vi "Host.vi"() -> ()   [LabVIEW 2019]
uses:
  <vilib>/Utility/Variable/NI_VariableUtilities.lvlib
  <vilib>/Utility/file.llb/Write Delimited Spreadsheet (DBL).vi
  <vilib>/Utility/file.llb/Read Delimited Spreadsheet (DBL).vi
panel:
  out "Rounds":i32
  in  "Load Path":bool
  in  "Save Path":bool
  out "z ls error":T1
  out "z en error":T1
  out "x ls error":T1
  out "x en error":T1
  in  "tLength":i32=15000
  in  "t0":i32=7500
  out "X LS (mm)":dbl[](graph)
  out "Z LS (mm)":dbl[](graph)
  out "LS Error X  (um)":dbl[](graph)
  out "EN Error X  (um)":dbl[](graph)
  out "LS Error Z  (um)":dbl[](graph)
  out "EN Error Z  (um)":dbl[](graph)
  in  "Save 2 txt":bool caption="Save ILC"
  out "Z EN (mm)":dbl[](graph)
  out "X EN (mm)":dbl[](graph)
  in  "Load data":bool caption="Save ILC"
  in  "Stop Host":bool
  in  "Generate Path":bool
  out "Position Command X (mm)":dbl[](graph)
  out "Position Command Z (mm)":dbl[](graph)
  in  "CLEAR X":bool
  in  "CLEAR Z":bool
  in  "ADD X":bool
  in  "ADD Z":bool
  in  "Time (s)":dbl=30.0 format="%#_13g"
  in  "Sample Rate (Hz)":dbl=1000.0 format="%#_13g"
  in  "Tab Control":enum32{"Const", "Ramp", "Chirp", "Sin", "Cos"}(tab)
  in  "Constant Value (mm)":dbl format="%#_13g"
  in  "Ramp Value (mm)":dbl=-10.0 format="%#_13g"
  in  "Chirp  Amp (mm)":dbl=50.0
  in  "Initial Frequency (Hz)":dbl
  in  "Final Frequency (Hz)":dbl=50.0
  in  "Decay":bool=TRUE
  in  "Sin  Amp (mm)":dbl=-50.0
  in  "Sin Periods (s)":dbl=15.0
  in  "Cos  Amp (mm)":dbl=50.0
  in  "Cos Periods (s)":dbl=15.0
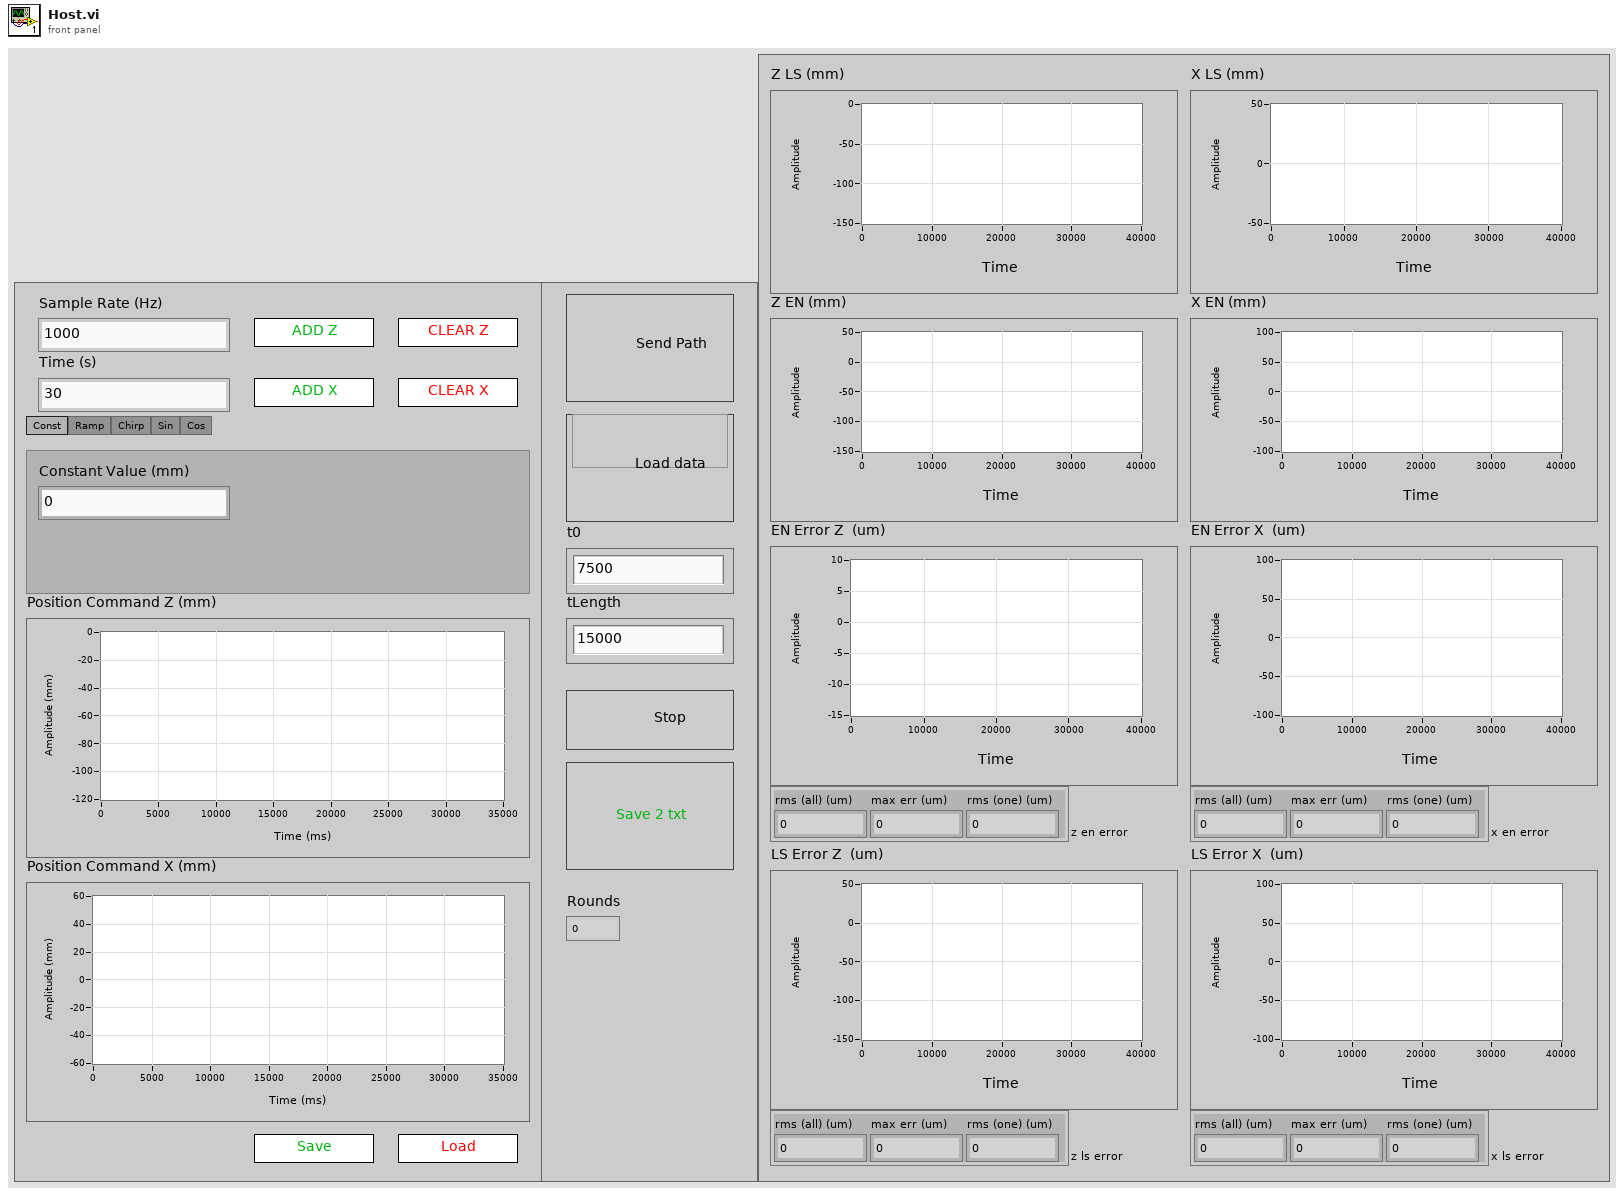
[diagram p1: front panel]
types:
  T1 = cluster{"rms (all) (um)":dbl, "max err (um)":dbl, "rms (one) (um)":dbl}
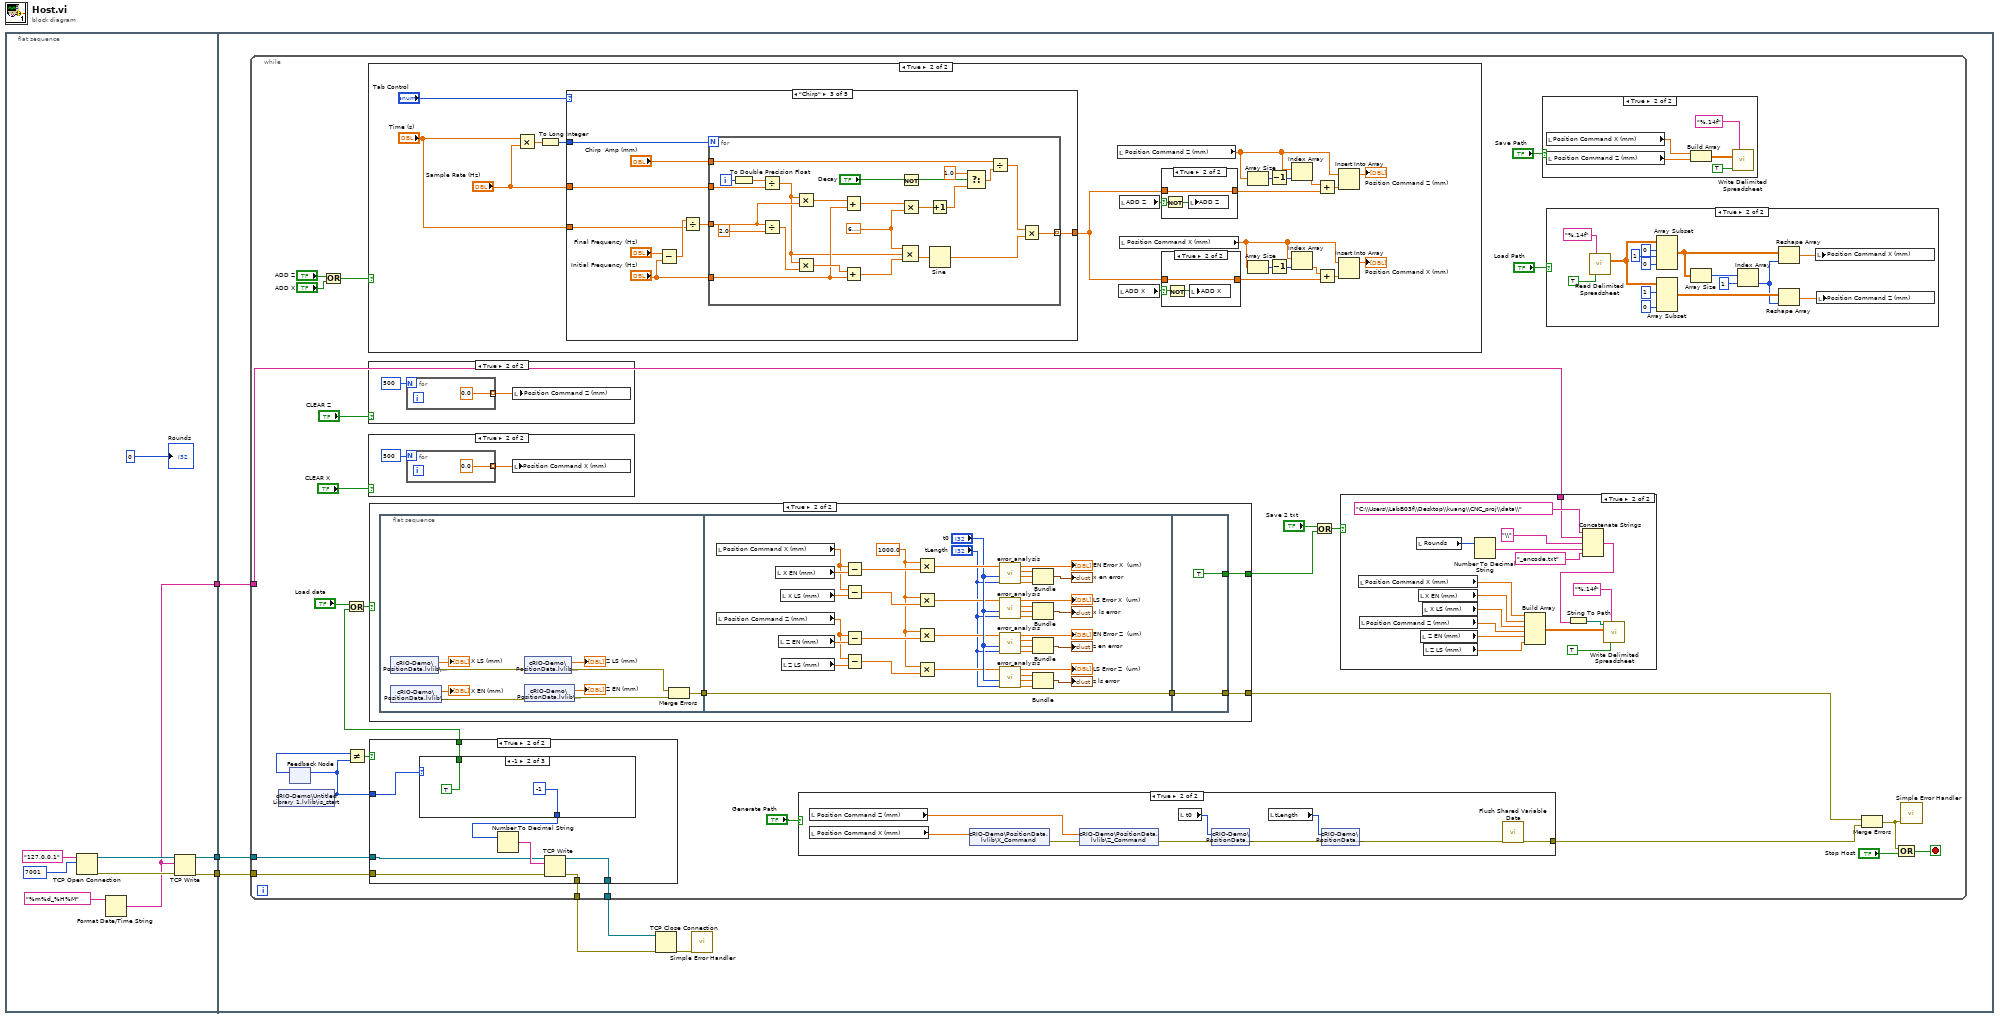
[diagram p0: block diagram]
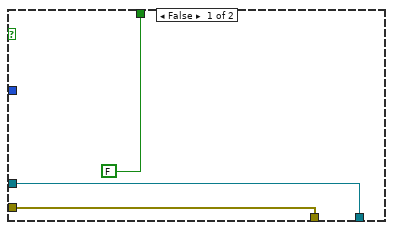
[diagram p2: hidden frame]
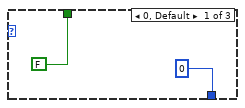
[diagram p3: hidden frame]
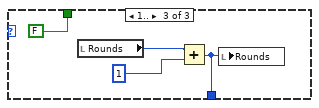
[diagram p4: hidden frame]
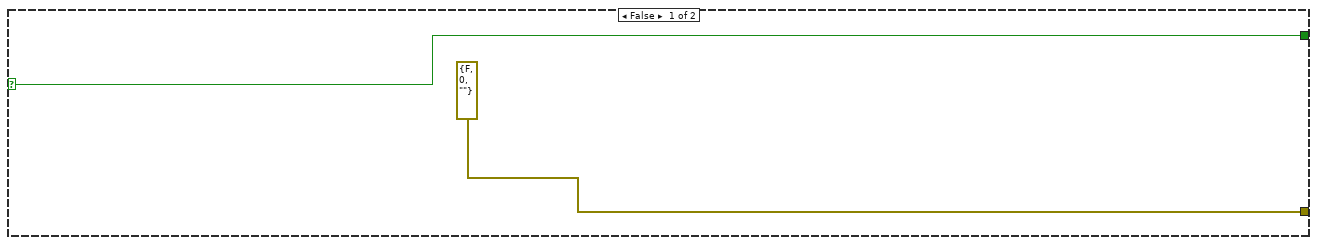
[diagram p8: hidden frame]
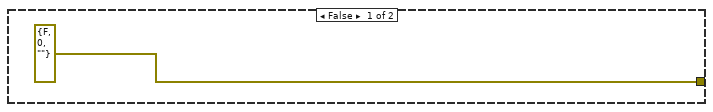
[diagram p9: hidden frame]
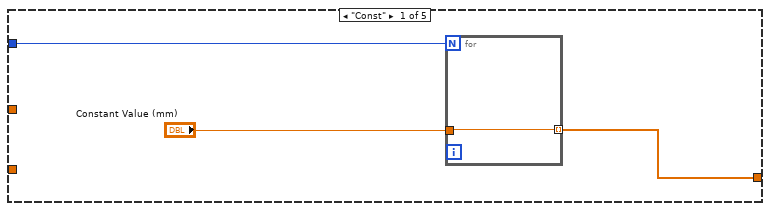
[diagram p13: hidden frame]
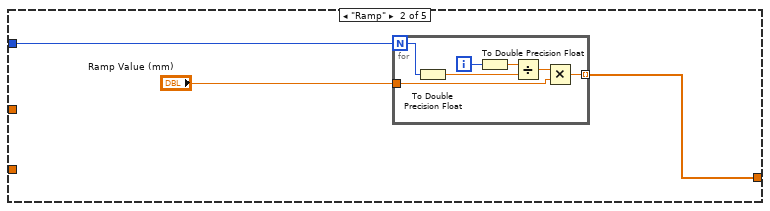
[diagram p14: hidden frame]
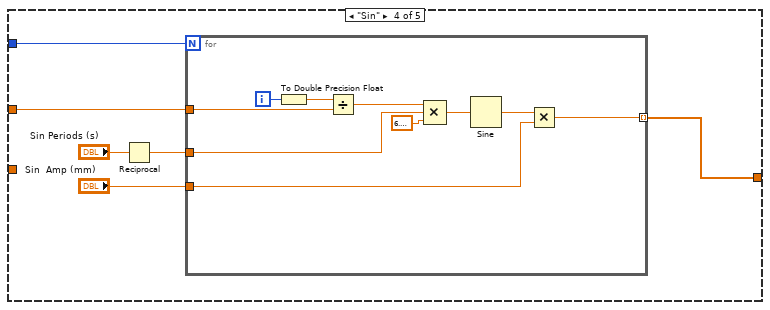
[diagram p15: hidden frame]
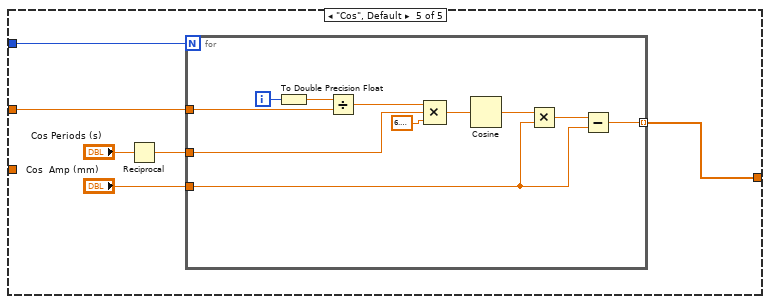
[diagram p16: hidden frame]
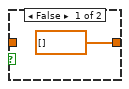
[diagram p17: hidden frame]
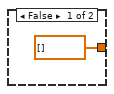
[diagram p18: hidden frame]
diagram:
  n1 = flat-sequence {
    tunnel: [w6] -> w3
    tunnel: [w5] -> w2
    tunnel: [w4] -> w1
    tunnel: w3 -> [w18]
    tunnel: w2 -> [w17]
    tunnel: w1 -> [w13]
    frame #0 {
      n2 = TCP Open Connection(address="127.0.0.1", remote port or service name=7001) -> (connection ID=w9:refnum<k5>, error out=w8:errorcluster)  [unwired: 3 in]
      n3 = Format Date/Time String(time format string (%c)="%m%d_%H%M") -> (date/time string=w4:string)  [unwired: 2 in]
      n4 = TCP Write(connection ID=w9, data in=w4, error in (no error)=w8) -> (connection ID out=w6:refnum<k5>, error out=w5:errorcluster)  [unwired: 1 in, 1 out]
      "Rounds" <- 0
    }
    frame #1 {
      n5 = while {
        tunnel: w18 -> [w29]
        tunnel: w17 -> [w28]
        tunnel: [w27] -> w16
        tunnel: [w26] -> w15
        tunnel: w13 -> [w25]
        stop <- w36 stop-if-true
        n6 = shared-variable "cRIO-Demo\\Untitled Library 1.lvlib\\is_start"() -> (w32:i16)  [unwired: 1 in, 1 out]
        n7 = feedback-in #1(w32) -> ()
        n8 = feedback #1() -> (w31:i16)  [unwired: 1 in]
        n9 = Or(x="ADD Z", y="ADD X") -> (x .or. y?=w43:bool)
        n10 = Not Equal?(x=w31, y=w32) -> (x != y?=w33:bool)
        n11 = case shown="True" w43 {
          frame False {
          }
          frame True {
            n12 = Multiply(x="Time (s)", y="Sample Rate (Hz)") -> (x*y=w179:dbl)
            n13 = To Long Integer(number=w179) -> (32bit integer=w178:i32)
            n14 = case shown="\"Chirp\"" "Tab Control" {
              tunnel: w178 -> [w197 w201 w217 w244 w263]
              tunnel: [w195 w199 w213 w243 w259] -> w175
              tunnel: "Sample Rate (Hz)" -> [_ _ w214 w242 w258]
              tunnel: "Time (s)" -> [_ _ w210 _ _]
              frame "Const" {
                n15 = for {
                  N: w197 -> [_]
                  tunnel: "Constant Value (mm)" -> [w198]
                  tunnel: [w198] -> w195 mode=indexing
                }
              }
              frame "Ramp" {
                n16 = for {
                  N: w201 -> [w204]
                  tunnel: [w206] -> w199 mode=indexing
                  tunnel: "Ramp Value (mm)" -> [w205]
                  i -> [w203]
                  n17 = To Double Precision Float(number=w204) -> (double precision float=w207:dbl)
                  n18 = To Double Precision Float(number=w203) -> (double precision float=w208:dbl)
                  n19 = Divide(x=w208, y=w207) -> (x/y=w202:dbl)
                  n20 = Multiply(x=w202, y=w205) -> (x*y=w206:dbl)
                }
              }
              frame "Chirp" {
                n21 = Subtract(x="Final Frequency (Hz)", y="Initial Frequency (Hz)") -> (x-y=w211:dbl)
                n22 = Divide(x=w211, y=w210) -> (x/y=w209:dbl)
                n23 = for {
                  N: w217 -> [_]
                  tunnel: "Chirp  Amp (mm)" -> [w218]
                  tunnel: [w236] -> w213 mode=indexing
                  tunnel: w209 -> [w227]
                  tunnel: w214 -> [w235]
                  tunnel: "Initial Frequency (Hz)" -> [w231]
                  i -> [w241]
                  w223 = 6.283185307179586
                  n24 = To Double Precision Float(number=w241) -> (double precision float=w240:dbl)
                  n25 = Divide(x=w240, y=w235) -> (x/y=w225:dbl)
                  n26 = Divide(x=w227, y=2.0) -> (x/y=w233:dbl)
                  n27 = Multiply(x=w225, y=w227) -> (x*y=w232:dbl)
                  n28 = Multiply(x=w225, y=w233) -> (x*y=w234:dbl)
                  n29 = Add(x=w232, y=w231) -> (x+y=w224:dbl)
                  n30 = Add(x=w234, y=w231) -> (x+y=w226:dbl)
                  n31 = Not(x="Decay") -> (.not. x?=w228:bool)
                  n32 = Multiply(x=w224, y=w223) -> (x*y=w230:dbl)
                  n33 = Compound Arithmetic op=MULTIPLY(w223, w225, w226) -> (w239:dbl)
                  n34 = Increment(x=w230) -> (x+1=w222:dbl)
                  n35 = Sine(x=w239) -> (sin(x)=w237:dbl)
                  n36 = Select(t=1.0, s=w228, f=w222) -> (s? t:f=w220:dbl)
                  n37 = Divide(x=w218, y=w220) -> (x/y=w221:dbl)
                  n38 = Multiply(x=w221, y=w237) -> (x*y=w236:dbl)
                }
              }
              frame "Sin" {
                n39 = Reciprocal(x="Sin Periods (s)") -> (1/x=w245:dbl)
                n40 = for {
                  N: w244 -> [_]
                  tunnel: [w249] -> w243 mode=indexing
                  tunnel: "Sin  Amp (mm)" -> [w252]
                  tunnel: w245 -> [w250]
                  tunnel: w242 -> [w248]
                  i -> [w251]
                  n41 = To Double Precision Float(number=w251) -> (double precision float=w255:dbl)
                  n42 = Divide(x=w255, y=w248) -> (x/y=w254:dbl)
                  n43 = Compound Arithmetic op=MULTIPLY(w254, w250, 6.283185307179586) -> (w257:dbl)
                  n44 = Sine(x=w257) -> (sin(x)=w253:dbl)
                  n45 = Multiply(x=w253, y=w252) -> (x*y=w249:dbl)
                }
              }
              frame "Cos", Default {
                n46 = Reciprocal(x="Cos Periods (s)") -> (1/x=w260:dbl)
                n47 = for {
                  N: w263 -> [_]
                  tunnel: [w268] -> w259 mode=indexing
                  tunnel: "Cos  Amp (mm)" -> [w267]
                  tunnel: w260 -> [w265]
                  tunnel: w258 -> [w264]
                  i -> [w266]
                  n48 = To Double Precision Float(number=w266) -> (double precision float=w272:dbl)
                  n49 = Divide(x=w272, y=w264) -> (x/y=w271:dbl)
                  n50 = Compound Arithmetic op=MULTIPLY(w271, w265, 6.283185307179586) -> (w274:dbl)
                  n51 = Cosine(x=w274) -> (cos(x)=w270:dbl)
                  n52 = Multiply(x=w270, y=w267) -> (x*y=w269:dbl)
                  n53 = Subtract(x=w269, y=w267) -> (x-y=w268:dbl)
                }
              }
            }
            n54 = local read "Position Command Z (mm)"() -> (w190:dbl[])
            n55 = local read "ADD X"() -> (w181:bool)
            n56 = local read "ADD Z"() -> (w182:bool)
            n57 = local read "Position Command X (mm)"() -> (w183:dbl[])
            n58 = case shown="True" w182 {
              selector: w182 -> [_ w277]
              tunnel: w175 -> [_ w278]
              tunnel: [dbl[] [] w278] -> w189
              frame False {
              }
              frame True {
                n59 = Not(x=w277) -> (.not. x?=w276:bool)
                n60 = local write "ADD Z"(w276) -> ()
              }
            }
            n61 = case shown="True" w181 {
              selector: w181 -> [_ w281]
              tunnel: [dbl[] [] w282] -> w184
              tunnel: w175 -> [_ w282]
              frame False {
              }
              frame True {
                n62 = Not(x=w281) -> (.not. x?=w280:bool)
                n63 = local write "ADD X"(w280) -> ()
              }
            }
            n64 = Array Size(array=w190) -> (size(s)=w194:i32)
            n65 = Array Size(array=w183) -> (size(s)=w188:i32)
            n66 = Decrement(x=w194) -> (x-1=w193:i32)
            n67 = Decrement(x=w188) -> (x-1=w187:i32)
            n68 = Index Array(array=w190, index=w193) -> (element=w192:dbl)
            n69 = Index Array(array=w183, index=w187) -> (element=w186:dbl)
            n70 = Add(x=w192, y=w189) -> (x+y=w191:dbl[])
            n71 = Add(x=w186, y=w184) -> (x+y=w185:dbl[])
            n72 = Insert Into Array(array=w190, new element=w191) -> (→"Position Command Z (mm)":dbl[])  [unwired: 1 in]
            n73 = Insert Into Array(array=w183, new element=w185) -> (→"Position Command X (mm)":dbl[])  [unwired: 1 in]
          }
        }
        n74 = case shown="True" "CLEAR Z" {
          frame False {
          }
          frame True {
            n75 = for {
              N: 500 -> [_]
              tunnel: [0.0 ("element")] -> w171 mode=indexing
            }
            n76 = local write "Position Command Z (mm)"(w171) -> ()
          }
        }
        n77 = case shown="True" "CLEAR X" {
          frame False {
          }
          frame True {
            n78 = for {
              N: 500 -> [_]
              tunnel: [0.0 ("element")] -> w168 mode=indexing
            }
            n79 = local write "Position Command X (mm)"(w168) -> ()
          }
        }
        n80 = case shown="True" w33 {
          tunnel: w32 -> [_ w52]
          tunnel: [w46 w55] -> w27
          tunnel: [w47 w54] -> w26
          tunnel: [FALSE w51] -> w22
          tunnel: w29 -> [w46 w50]
          tunnel: w28 -> [w47 w49]
          frame False {
          }
          frame True {
            n81 = case shown="-1" w52 {
              tunnel: [0 -1 w62] -> w53
              tunnel: [FALSE TRUE FALSE] -> w51
              frame 0, Default {
              }
              frame -1 {
              }
              frame 1.. {
                n82 = local read "Rounds"() -> (w63:i32)
                n83 = Add(x=w63, y=1) -> (x+y=w62:i32)
                n84 = local write "Rounds"(w62) -> ()
              }
            }
            n85 = Number To Decimal String(number=w53) -> (decimal integer string=w56:string)  [unwired: 1 in]
            n86 = TCP Write(connection ID=w50, data in=w56, error in (no error)=w49) -> (connection ID out=w55:refnum<k5>, error out=w54:errorcluster)  [unwired: 1 in, 1 out]
          }
        }
        n87 = Or(x="Load data", y=w22) -> (x .or. y?=w24:bool)
        n88 = case shown="True" w24 {
          selector: w24 -> [w102 _]
          tunnel: [errorcluster {"status"=FALSE, "code"=0, "source"=""} ("error IO") w107] -> w38
          tunnel: [w102 w104] -> w19
          frame False {
          }
          frame True {
            n89 = flat-sequence {
              tunnel: [w109] -> w106
              tunnel: w106 -> [w154]
              tunnel: [w154] -> w105
              tunnel: [w156] -> w107
              tunnel: w105 -> [w156]
              tunnel: [TRUE] -> w104
              frame #0 {
                n90 = shared-variable "cRIO-Demo\\PositionData.lvlib\\X_LS"() -> (→"X LS (mm)":dbl[], error out=w112:errorcluster)  [unwired: 1 in]
                n91 = shared-variable "cRIO-Demo\\PositionData.lvlib\\X_EN"() -> (→"X EN (mm)":dbl[], error out=w116:errorcluster)  [unwired: 1 in]
                n92 = shared-variable "cRIO-Demo\\PositionData.lvlib\\Z_LS"(error in=w112) -> (→"Z LS (mm)":dbl[], error out=w108:errorcluster)
                n93 = shared-variable "cRIO-Demo\\PositionData.lvlib\\Z_EN"(error in=w116) -> (→"Z EN (mm)":dbl[], error out=w110:errorcluster)
                n94 = Merge Errors(w108, w110) -> (w109:errorcluster)
              }
              frame #1 {
                w143 = 1000.0
                n95 = local read "Position Command X (mm)"() -> (w149:dbl[])
                n96 = local read "Position Command Z (mm)"() -> (w148:dbl[])
                n97 = local read "X EN (mm)"() -> (w153:dbl[])
                n98 = local read "Z EN (mm)"() -> (w151:dbl[])
                n99 = local read "X LS (mm)"() -> (w152:dbl[])
                n100 = local read "Z LS (mm)"() -> (w150:dbl[])
                n101 = Subtract(x=w149, y=w153) -> (x-y=w147:dbl[])
                n102 = Subtract(x=w149, y=w152) -> (x-y=w146:dbl[])
                n103 = Subtract(x=w148, y=w151) -> (x-y=w145:dbl[])
                n104 = Subtract(x=w148, y=w150) -> (x-y=w144:dbl[])
                n105 = Multiply(x=w143, y=w147) -> (x*y=w142:dbl[])
                n106 = Multiply(x=w143, y=w146) -> (x*y=w120:dbl[])
                n107 = Multiply(x=w143, y=w145) -> (x*y=w119:dbl[])
                n108 = Multiply(x=w143, y=w144) -> (x*y=w118:dbl[])
                n109 = call "error_analysis.vi"("tLength"="tLength", "t0"="t0", "data in (um)"=w142) -> ("rms (one) (um)"=w137:dbl, "max err (um)"=w138:dbl, "rms (all) (um)"=w139:dbl, "data out (um)"=→"EN Error X  (um)":dbl[])  [unwired: 5 in]
                n110 = call "error_analysis.vi"("tLength"="tLength", "t0"="t0", "data in (um)"=w120) -> ("rms (one) (um)"=w133:dbl, "max err (um)"=w134:dbl, "rms (all) (um)"=w135:dbl, "data out (um)"=→"LS Error X  (um)":dbl[])  [unwired: 5 in]
                n111 = call "error_analysis.vi"("tLength"="tLength", "t0"="t0", "data in (um)"=w119) -> ("rms (one) (um)"=w129:dbl, "max err (um)"=w130:dbl, "rms (all) (um)"=w131:dbl, "data out (um)"=→"EN Error Z  (um)":dbl[])  [unwired: 5 in]
                n112 = call "error_analysis.vi"("tLength"="tLength", "t0"="t0", "data in (um)"=w118) -> ("rms (one) (um)"=w126:dbl, "max err (um)"=w127:dbl, "rms (all) (um)"=w128:dbl, "data out (um)"=→"LS Error Z  (um)":dbl[])  [unwired: 5 in]
                n113 = Bundle("rms (all) (um)"=w139, "max err (um)"=w138, "rms (one) (um)"=w137) -> (→"x en error":T1)  [unwired: 1 in]
                n114 = Bundle("rms (all) (um)"=w135, "max err (um)"=w134, "rms (one) (um)"=w133) -> (→"x ls error":T1)  [unwired: 1 in]
                n115 = Bundle("rms (all) (um)"=w131, "max err (um)"=w130, "rms (one) (um)"=w129) -> (→"z en error":T1)  [unwired: 1 in]
                n116 = Bundle("rms (all) (um)"=w128, "max err (um)"=w127, "rms (one) (um)"=w126) -> (→"z ls error":T1)  [unwired: 1 in]
              }
              frame #2 {
              }
            }
          }
        }
        n117 = case shown="True" "Generate Path" {
          tunnel: [errorcluster {"status"=FALSE, "code"=0, "source"=""} ("error IO") w163] -> w39
          frame False {
          }
          frame True {
            n118 = local read "Position Command Z (mm)"() -> (w164:dbl[])
            n119 = local read "Position Command X (mm)"() -> (w166:dbl[])
            n120 = shared-variable "cRIO-Demo\\PositionData.lvlib\\X_Command"(w166) -> (error out=w165:errorcluster)  [unwired: 1 in]
            n121 = shared-variable "cRIO-Demo\\PositionData.lvlib\\Z_Command"(w164, error in=w165) -> (error out=w161:errorcluster)
            n122 = local read "t0"() -> (w159:i32)
            n123 = shared-variable "cRIO-Demo\\PositionData.lvlib\\t0"(w159, error in=w161) -> (error out=w162:errorcluster)
            n124 = local read "tLength"() -> (w158:i32)
            n125 = shared-variable "cRIO-Demo\\PositionData.lvlib\\tL"(w158, error in=w162) -> (error out=w160:errorcluster)
            n126 = call <vilib>:"Flush Shared Variable Data.vi"("error in (no error)"=w160) -> ("error out"=w163:errorcluster)  [unwired: 10 in]
          }
        }
        n127 = Or(x="Save 2 txt", y=w19) -> (x .or. y?=w21:bool)
        n128 = case shown="True" w21 {
          tunnel: w25 -> [_ w85]
          frame False {
          }
          frame True {
            n129 = local read "Position Command X (mm)"() -> (w99:dbl[])
            n130 = local read "Position Command Z (mm)"() -> (w96:dbl[])
            n131 = local read "Rounds"() -> (w90:i32)
            n132 = local read "X EN (mm)"() -> (w98:dbl[])
            n133 = local read "Z EN (mm)"() -> (w95:dbl[])
            n134 = local read "X LS (mm)"() -> (w97:dbl[])
            n135 = local read "Z LS (mm)"() -> (w94:dbl[])
            n136 = Number To Decimal String(number=w90) -> (decimal integer string=w89:string)  [unwired: 1 in]
            n137 = Build Array(w99, w98, w97, w96, w95, w94) -> (w101:dbl[][])
            n138 = Concatenate Strings("C:\\Users\\LabB03f\\Desktop\\kuang\\CNC_proj\\data\\", w85, "\\", w89, "_encode.txt") -> (w86:string)
            n139 = String To Path(string=w86) -> (path=w92:path)
            n140 = call-poly <vilib>:"Write Delimited Spreadsheet.vi"("file path (dialog if empty)"=w92, "format (%.3f)"="%.14f", "2D data"=w101, "transpose? (no:F)"=TRUE ("transpose? (F)")) -> ()  [unwired: 10 in, 2 out]
          }
        }
        n141 = case shown="True" "Save Path" {
          frame False {
          }
          frame True {
            n142 = local read "Position Command X (mm)"() -> (w82:dbl[])
            n143 = local read "Position Command Z (mm)"() -> (w81:dbl[])
            n144 = Build Array(w82, w81) -> (w80:dbl[][])
            n145 = call-poly <vilib>:"Write Delimited Spreadsheet.vi"("format (%.3f)"="%.14f", "2D data"=w80, "transpose? (no:F)"=TRUE ("transpose? (F)")) -> ()  [unwired: 11 in, 2 out]
          }
        }
        n146 = case shown="True" "Load Path" {
          frame False {
          }
          frame True {
            n147 = call-poly <vilib>:"Read Delimited Spreadsheet.vi"("format (%.3f)"="%.14f", "transpose? (F)"=TRUE) -> ("all rows"=w77:dbl[][])  [unwired: 8 in, 5 out]
            n148 = Array Subset(array=w77, index (row)=0 ("index"), length (row)=1 ("length"), index (col)=0 ("index")) -> (w69:dbl[][])  [unwired: 1 in]
            n149 = Array Subset(array=w77, index (row)=1 ("index"), index (col)=0 ("index")) -> (w68:dbl[][])  [unwired: 2 in]
            n150 = Array Size(array=w69) -> (size(s)=w71:i32[])
            n151 = Index Array(array=w71, index=1) -> (element=w67:i32)
            n152 = Reshape Array(w69, w67) -> (w66:dbl[])
            n153 = Reshape Array(w68, w67) -> (w65:dbl[])
            n154 = local write "Position Command X (mm)"(w66) -> ()
            n155 = local write "Position Command Z (mm)"(w65) -> ()
          }
        }
        n156 = Merge Errors(w38, w39) -> (w30:errorcluster)
        n157 = Compound Arithmetic op=OR(w30, "Stop Host") -> (w36:bool)
        n158 = call <vilib>:"Simple Error Handler.vi"("error in (no error)"=w30) -> ()  [unwired: 4 in, 5 out]
      }
      n159 = TCP Close Connection(connection ID=w16, error in (no error)=w15) -> (error out=w14:errorcluster)  [unwired: 1 in, 1 out]
      n160 = call <vilib>:"Simple Error Handler.vi"("error in (no error)"=w14) -> ()  [unwired: 4 in, 5 out]
    }
  }
